vi "Main_UI Gb.vi"() -> ()   [LabVIEW 2019]
panel:
  out "Main Page UI Ref":variant
  out "Image Glb":variant
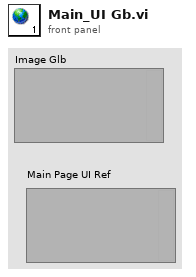
[diagram p1: front panel]
diagram:
